vi "DisConnect.vi"(8 "error in (no error)":errorcluster, 11 "Red Pitaya in":refnum<class "Red Pitaya.lvclass">) -> (0 "error out":errorcluster, 3 "Red Pitaya out":refnum<class "Red Pitaya.lvclass">)   [LabVIEW 2015, in "Red Pitaya.lvclass"]
uses:
  Red Pitaya.lvclass
  Red Pitaya.lvclass/Red Pitaya.ctl
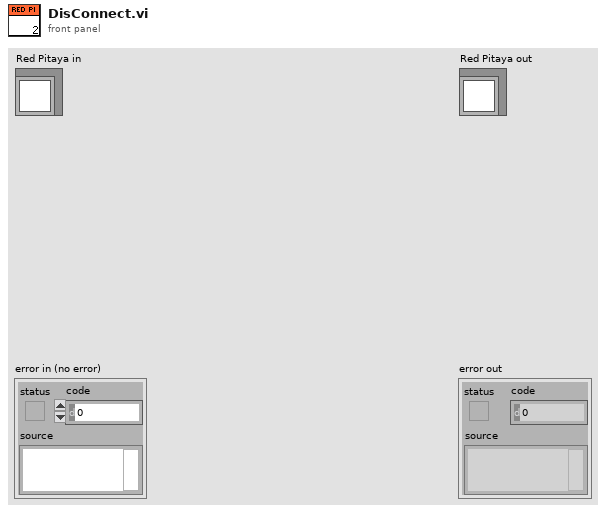
[diagram p1: front panel]
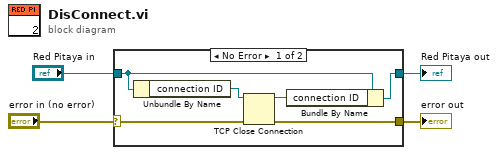
[diagram p0: block diagram]
diagram:
  n1 = case shown="No Error" "error in (no error)" {
    selector: "error in (no error)" -> [w7 w12]
    tunnel: [w6 w12] -> w3
    tunnel: [w9 w11] -> w1
    tunnel: "Red Pitaya in" -> [w10 w11]
    frame No Error {
      n2 = Unbundle By Name(w10) -> ("connection ID"=w5:refnum<k5>)
      n3 = TCP Close Connection(connection ID=w5, error in (no error)=w7) -> (connection ID out=w8:refnum<k5>, error out=w6:errorcluster)  [unwired: 1 in]
      n4 = Bundle By Name(cluster=w10, "connection ID"=w8) -> (w9:refnum<class "Red Pitaya.lvclass">)
    }
    frame Error {
    }
  }
  "error out" <- w3
  "Red Pitaya out" <- w1
